vi "AssertDisabled.vi"(0 "VI Reference In":refnum<vi>, 1 "Label":string, 2 "delimiter (>>)":string=">>", 3 "Assert Only? (F)":bool, 5 "Control Path":string, 11 "Error In":errorcluster, 12 "Assert Interval(10 ms)":u32=10, 13 "Timeout(5 sec)":dbl=5.0) -> (4 "VI Reference Out":refnum<vi>, 15 "Error Out":errorcluster)   [LabVIEW 2016, in "Drona.lvlib" / "AssertControlDisable.lvlib"]
doc: "Asserts the state of controls.\n\nThe input control name is given as a string , incase of path, use delimiters inbetween the path."
uses:
  AssertControlDisable.lvlib
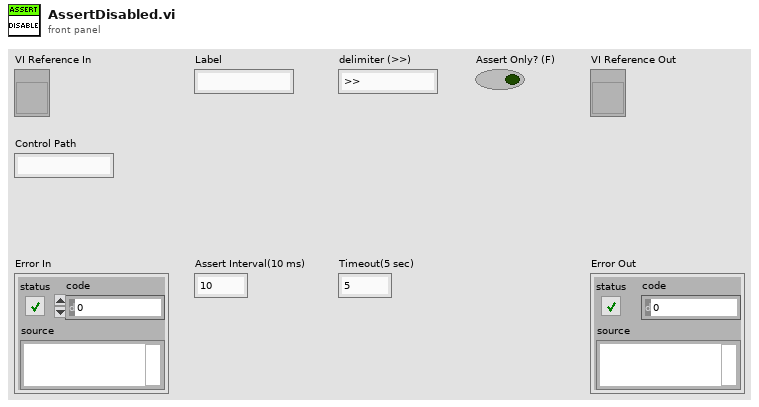
[diagram p1: front panel]
types:
  T1 = enum8{"Enabled", "Disabled", "Disabled and Grayed Out"}
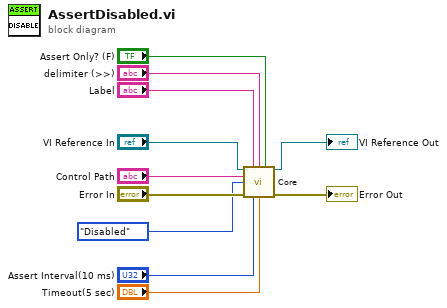
[diagram p0: block diagram]
diagram:
  n1 = call "Core.vi"("VI Reference In"="VI Reference In", "Label"="Label", "delimiter (>>)"="delimiter (>>)", "Assert Only? (F)"="Assert Only? (F)", "Control Path"="Control Path", "Disabled"=T1."Disabled", "Error In"="Error In", "Assert Interval(10 ms)"="Assert Interval(10 ms)", "Timeout(5 sec)"="Timeout(5 sec)") -> ("VI Reference Out"=→"VI Reference Out":refnum<vi>, "Error Out"=→"Error Out":errorcluster)  [unwired: 5 in]
